vi "Transmit Data.vi"(8 "error in (no error)":errorcluster, 10 "Data":i32[](array[numeric]), 11 "RP Instrument in":refnum<class "RP Instrument.lvclass">) -> (0 "error out":errorcluster, 3 "RP Instrument out":refnum<class "RP Instrument.lvclass">)   [LabVIEW 2016, in "RP Instrument.lvclass"]
uses:
  RP Instrument.lvclass
  RP Instrument.lvclass/RP Instrument.ctl
  RP Communicator/RP Communicator.lvclass
panel:
  out "Wait cycle counter":i32
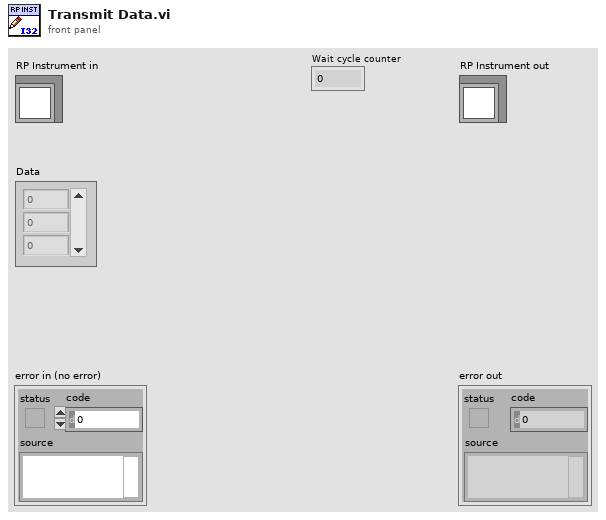
[diagram p1: front panel]
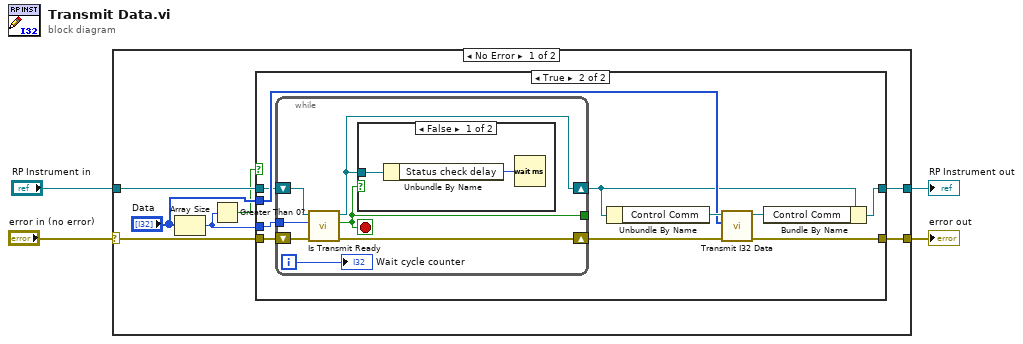
[diagram p0: block diagram]
diagram:
  n1 = case shown="No Error" "error in (no error)" {
    selector: "error in (no error)" -> [w7 w34]
    tunnel: [w9 w34] -> w3
    tunnel: [w11 w33] -> w1
    tunnel: "RP Instrument in" -> [w8 w33]
    frame No Error {
      n2 = Array Size(array="Data") -> (size(s)=w6:i32)
      n3 = Greater Than 0?(x=w6) -> (x > 0?=w5:bool)
      n4 = case shown="True" w5 {
        tunnel: [w12 w21] -> w11
        tunnel: "Data" -> [_ w20]
        tunnel: [w13 w19] -> w9
        tunnel: w8 -> [w12 w18]
        tunnel: w6 -> [_ w16]
        tunnel: w7 -> [w13 w15]
        frame False {
        }
        frame True {
          n5 = while {
            shift-right: [w28] -> w14
            shift-left: w15 -> [w29]
            shift-right: [w25] -> w17
            shift-left: w18 -> [w30]
            tunnel: [w27] -> _
            tunnel: w16 -> [w26]
            i -> [w24]
            stop <- w27 stop-if-true
            n6 = call-dynamic "Is Transmit Ready.vi"("error in (no error)"=w29, "Samples to transmit"=w26, "RP Instrument in"=w30) -> ("error out"=w28:errorcluster, "Transmit Ready"=w27:bool, "RP Instrument out"=w25:refnum<class "RP Instrument.lvclass">)  [unwired: 5 in, 1 out]
            n7 = case shown="False" w27 {
              tunnel: w25 -> [w32 _]
              frame False {
                n8 = Unbundle By Name(w32) -> ("Status check delay"=w31:u32)
                n9 = Wait (ms)(milliseconds to wait=w31) -> ()  [unwired: 1 out]
              }
              frame True {
              }
            }
            "Wait cycle counter" <- w24
          }
          n10 = Unbundle By Name(w17) -> ("Control Comm"=w23:refnum<class "RP Communicator.lvclass">)
          n11 = call-dynamic "Transmit I32 Data.vi"("error in (no error)"=w14, "Data"=w20, "RP Communicator in"=w23) -> ("error out"=w19:errorcluster, "RP Communicator out"=w22:refnum<class "RP Communicator.lvclass">)  [unwired: 7 in]
          n12 = Bundle By Name(cluster=w17, "Control Comm"=w22) -> (w21:refnum<class "RP Instrument.lvclass">)
        }
      }
    }
    frame Error {
    }
  }
  "error out" <- w3
  "RP Instrument out" <- w1
